vi "Action Log Data.vi"(0 "VISA resource name":refnum<visa-resource-name>, 7 "Log Data (F: Logging OFF)":bool, 11 "error in (no error)":errorcluster) -> (4 "VISA resource name out":refnum<visa-resource-name>, 15 "error out":errorcluster)   [LabVIEW 2012, in "Lake Shore Cryotronics 218.lvlib"]
doc: "This VI turns data logging on and off."
uses:
  <instrlib>/Lake Shore Cryotronics 218/Lake Shore Cryotronics 218.lvlib
panel:
  # "Logging ON\nLogging OFF"
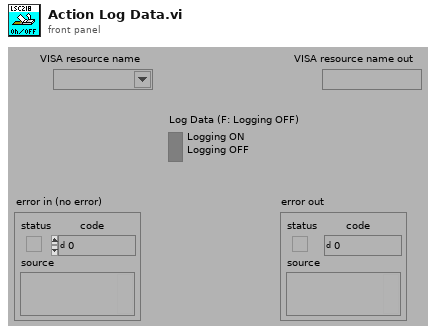
[diagram p1: front panel]
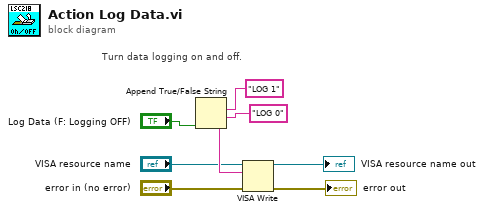
[diagram p0: block diagram]
diagram:
  # "Turn data logging on and off."
  n1 = Append True/False String(1:"Log Data (F: Logging OFF)", 2:"LOG 0", 3:"LOG 1") -> (0:w5:string)  [unwired: 1 in]
  n2 = VISA Write(VISA resource name="VISA resource name", write buffer=w5, error in (no error)="error in (no error)") -> (VISA resource name out=→"VISA resource name out":refnum<visa-resource-name>, error out=→"error out":errorcluster)  [unwired: 1 out]
